vi "Close.vi"(8 "error in (no error)":errorcluster, 11 "VICI Settings":T1 {"Pump Number" min=1.0 max=20.0 step=1.0}) -> (0 "error out":errorcluster, 3 "VICI Settings":T1 {"Pump Number" min=1.0 max=20.0 step=1.0})   [LabVIEW 2018, in "VICI M50.lvlib"]
uses:
  VICI M50.lvlib
  Settings Cluster.ctl
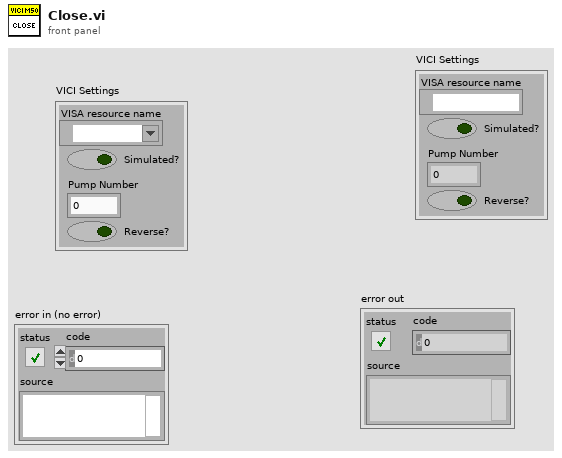
[diagram p1: front panel]
types:
  T1 = typedef "Settings Cluster.ctl" = cluster{"VISA resource name":refnum<visa-resource-name>, "Simulated?":bool, "Pump Number":dbl, "Reverse?":bool}
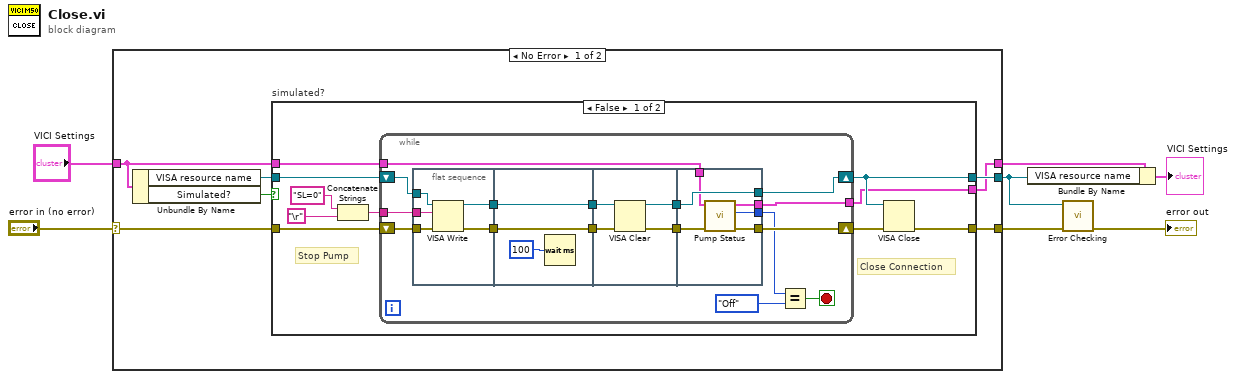
[diagram p0: block diagram]
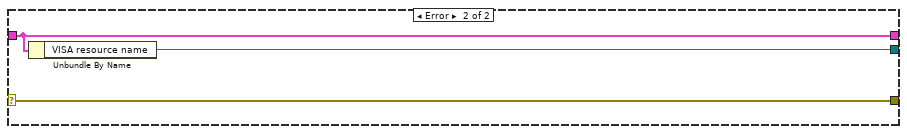
[diagram p3: hidden frame]
diagram:
  n1 = case shown="No Error" "error in (no error)" {
    selector: "error in (no error)" -> [w12 w64]
    tunnel: [w13 w64] -> w5
    tunnel: "VICI Settings" -> [w9 w62]
    tunnel: [w10 w63] -> w2
    tunnel: [w8 w62] -> w1
    frame No Error {
      n2 = Unbundle By Name(w9) -> ("VISA resource name"=w11:refnum<visa-resource-name>, "Simulated?"=w14:bool)
      n3 = case "simulated?" shown="False" w14 {
        tunnel: [w19 w61] -> w13
        tunnel: w11 -> [w18 w60]
        tunnel: w12 -> [w22 w61]
        tunnel: [w17 w60] -> w10
        tunnel: w9 -> [w16 w59]
        tunnel: [w15 w59] -> w8
        frame False {
          # "Close Connection"
          # "Stop Pump"
          n4 = Concatenate Strings("SL=0" ("string"), "\r") -> (w21:string)
          n5 = while {
            tunnel: w21 -> [w33]
            shift-right: [w32] -> w20
            shift-left: w22 -> [w34]
            shift-right: [w30] -> w17
            shift-left: w18 -> [w31]
            tunnel: w16 -> [w28]
            tunnel: [w27] -> w15
            stop <- w29 stop-if-true
            n6 = flat-sequence {
              tunnel: [w41] -> w40
              tunnel: [w42] -> w39
              tunnel: w34 -> [w45]
              tunnel: w33 -> [w44]
              tunnel: w31 -> [w43]
              tunnel: w40 -> [w48]
              tunnel: [w48] -> w38
              tunnel: w39 -> [w47]
              tunnel: [w47] -> w37
              tunnel: w38 -> [w52]
              tunnel: w37 -> [w51]
              tunnel: [w50] -> w36
              tunnel: [w49] -> w35
              tunnel: [w58] -> w30
              tunnel: [w56] -> w32
              tunnel: w36 -> [w57]
              tunnel: w35 -> [w58]
              tunnel: [w55] -> w26
              tunnel: w28 -> [w54]
              tunnel: [w53] -> w27
              frame #0 {
                n7 = VISA Write(VISA resource name=w43, write buffer=w44, error in (no error)=w45) -> (VISA resource name out=w41:refnum<visa-resource-name>, error out=w42:errorcluster)  [unwired: 1 out]
              }
              frame #1 {
                n8 = Wait (ms)(milliseconds to wait=u32 100) -> ()  [unwired: 1 out]
              }
              frame #2 {
                n9 = VISA Clear(VISA resource name=w52, error in (no error)=w51) -> (VISA resource name out=w49:refnum<visa-resource-name>, error out=w50:errorcluster)
              }
              frame #3 {
                n10 = call "Pump Status.vi"("error in (no error)"=w57, "VICI Settings In"=w54) -> ("error out"=w56:errorcluster, "Pump On?"=w55:enum16{"Off", "On", "Not Initialized"}, "VICI Settings Out"=w53:T1)  [unwired: 6 in, 1 out]
              }
            }
            n11 = Equal?(x=w26, y=enum16{"Off", "On", "Not Initialized"}."Off") -> (x = y?=w29:bool)
          }
          n12 = VISA Close(VISA resource name=w17, error in (no error)=w20) -> (error out=w19:errorcluster)
        }
        frame True {
        }
      }
    }
    frame Error {
      n13 = Unbundle By Name(w62) -> ("VISA resource name"=w63:refnum<visa-resource-name>)
    }
  }
  n14 = Bundle By Name(cluster=w1, "VISA resource name"=w2) -> (→"VICI Settings":T1)
  n15 = call "Error Checking.vi"("error in (no error)"=w5, "VISA resource name"=w2) -> ("error out"=→"error out":errorcluster)  [unwired: 7 in, 2 out]
